vi "averageofrandimnumber.vi"() -> ()   [LabVIEW 2015]
panel:
  out "Numeric":i32
  out "random_no":dbl
  out "average":dbl
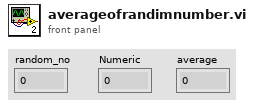
[diagram p1: front panel]
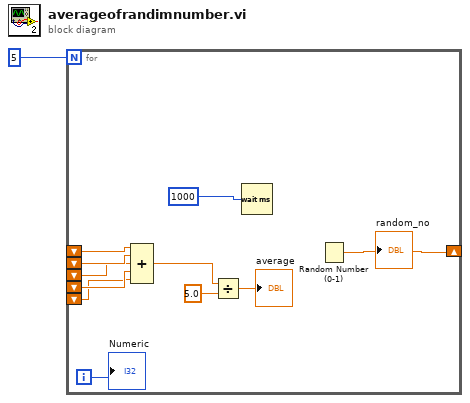
[diagram p0: block diagram]
diagram:
  n1 = for {
    N: 5 -> [_]
    shift-right: [w12] -> _
    shift-left: _ -> [w11]
    shift-left: _ -> [w10]
    shift-left: _ -> [w9]
    shift-left: _ -> [w8]
    shift-left: _ -> [w7]
    i -> [w3]
    n2 = Compound Arithmetic op=ADD(w11, w10, w9, w8, w7) -> (w6:dbl)
    n3 = Divide(x=w6, y=5.0) -> (x/y=→"average":dbl)
    n4 = Wait (ms)(milliseconds to wait=u32 1000 ("millisecond timer value")) -> ()  [unwired: 1 out]
    n5 = Random Number (0-1)() -> (number: 0 to 1=w12:dbl)
    "random_no" <- w12
    "Numeric" <- w3
  }
